vi "Fetch Measurement.vi"   [LabVIEW 2022 SP3, in "Agilent N934X Series.lvlib"]
doc: "This is a poly VI for fetch measurement VIs."
uses:
  <instrlib>/Agilent N934X Series/Agilent N934X Series.lvlib
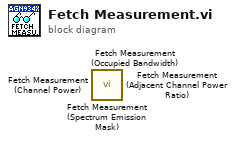
[diagram p0: block diagram]
diagram:
  n1 = call <instrlib>:"Fetch Measurement (Spectrum Emission Mask).vi"() -> ()  [unwired: 13 in, 3 out]
  n2 = call <instrlib>:"Fetch Measurement (Occupied Bandwidth).vi"() -> ()  [unwired: 12 in, 4 out]
  n3 = call <instrlib>:"Fetch Measurement (Channel Power).vi"() -> ()  [unwired: 12 in, 4 out]
  n4 = call <instrlib>:"Fetch Measurement (Adjacent Channel Power Ratio).vi"() -> ()  [unwired: 9 in, 7 out]
